vi "Create Voltage Output.vi"(8 "error in (no error)":errorcluster, 10 "Params":variant, 11 "NI Analog Output in":refnum<class "NI Analog Output.lvclass">) -> (0 "error out":errorcluster, 3 "NI Analog Output out":refnum<class "NI Analog Output.lvclass">)   [LabVIEW 2020, in "NI DAQmx.lvlib" / "NI Analog Output.lvclass"]
uses:
  NI Analog Output.lvclass
  D:/WSGitHub/RTFWK/Realization/NI DAQmx Base/NI DAQmx Base.lvclass
  NI DAQmx Base/TypeDefs/Channel Config.ctl
  <vilib>/DAQmx/create/channels.llb/DAQmx Create Channel (AO-Voltage-Basic).vi
  <vilib>/Utility/Data Type/NI_Data Type.lvlib
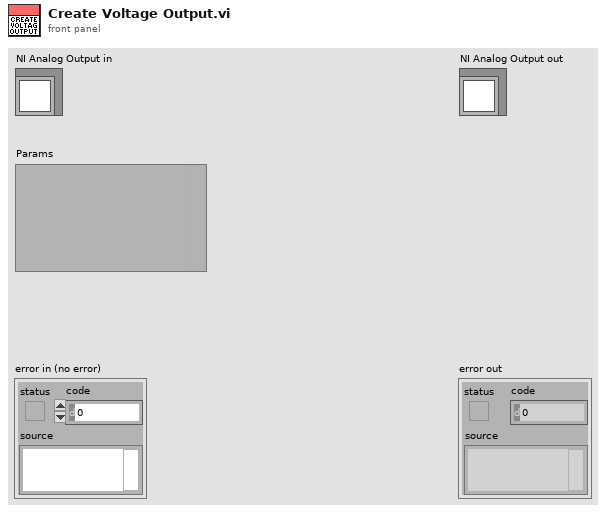
[diagram p1: front panel]
types:
  T1 = typedef "Channel Config.ctl" = cluster{"channels":string, "maximum value":dbl, "minimum value":dbl, "output terminal configuration":i32, "units":i32}
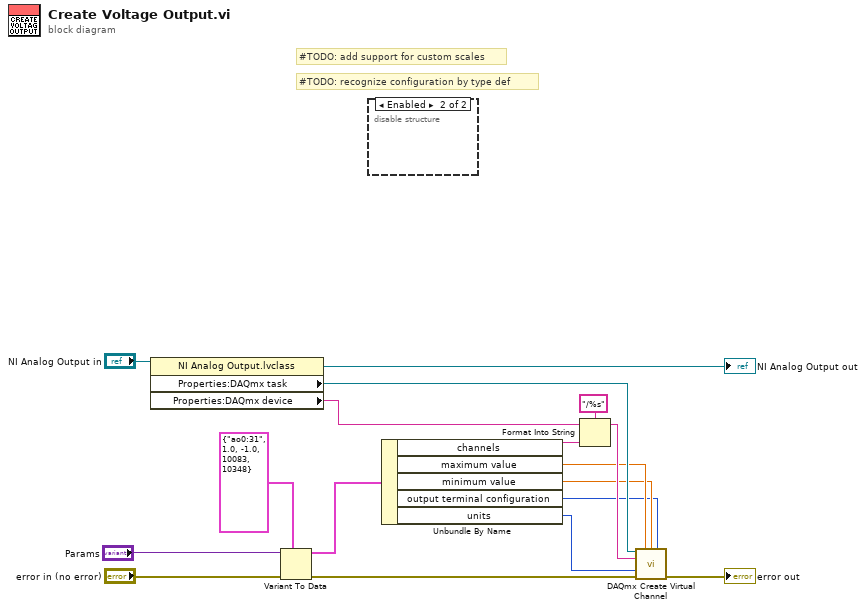
[diagram p0: block diagram]
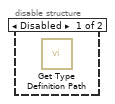
[diagram p2: hidden frame]
diagram:
  # "#TODO: add support for custom scales"
  # "#TODO: recognize configuration by type def"
  n1 = property class="NI Analog Output.lvclass"(reference="NI Analog Output in") -> (reference out=→"NI Analog Output out":refnum<class "NI Analog Output.lvclass">, "Properties:DAQmx task"=w11:refnum<k21>, "Properties:DAQmx device"=w12:tag)  [unwired: 1 in, 1 out]
  n2 = Variant To Data(error in="error in (no error)", type=T1 {"channels"="ao0:31", "maximum value"=1.0, "minimum value"=-1.0, "output terminal configuration"=10083, "units"=10348} ("Channel Config"), Variant="Params") -> (data=w3:T1, error out=w14:errorcluster)
  n3 = disable-structure shown="Enabled" {
    frame Disabled {
      n4 = call <vilib>:"Get Type Definition Path.vi"() -> ()  [unwired: 10 in, 2 out]
    }
    frame Enabled {
    }
  }
  n5 = Unbundle By Name(w3) -> ("channels"=w9:string, "maximum value"=w7:dbl, "minimum value"=w6:dbl, "output terminal configuration"=w5:i32, "units"=w4:i32)
  n6 = Format Into String(format string="/%s", initial string=w12, w9) -> (resulting string=w8:string)  [unwired: 1 in, 1 out]
  n7 = call-poly <vilib>:"DAQmx Create Virtual Channel.vi"("task in"=w11, "maximum value"=w7, "minimum value"=w6, "output terminal configuration"=w5, "physical channels"=w8, "units"=w4, "error in"=w14) -> ("error out"=→"error out":errorcluster)  [unwired: 7 in, 1 out]
